vi "Init_Camera.vi"(4 "Binning IN":u32, 6 "Use Cursors IN":bool, 8 "Image Handle IN":u32=99 caption="Image Handle", 9 "ROI Parameters":T2={"X start"=1, "X end"=1340, "X Binning/Grouping"=1, "Y start"=1, "Y end"=400, "Y Binning/Grouping"=1}, 10 "integration time [s]":dbl=0.5, 11 "Parameters IN":T1={"camera parameters"={"Camera Handle"=16842752, "Xdim"=1340, "Ydim"=400}, "error"={"status"=FALSE, "code"=0, "source"=""}, "Plot height [pixel]"=0.0, "Plot width [pixel]"=0.0}) -> (0 "Image Handle OUT":u32 caption="Image Handle", 3 "Parameters OUT":T1={"camera parameters"={"Camera Handle"=16842752, "Xdim"=1340, "Ydim"=400}, "error"={"status"=FALSE, "code"=0, "source"=""}, "Plot height [pixel]"=0.0, "Plot width [pixel]"=0.0})   [LabVIEW 2013]
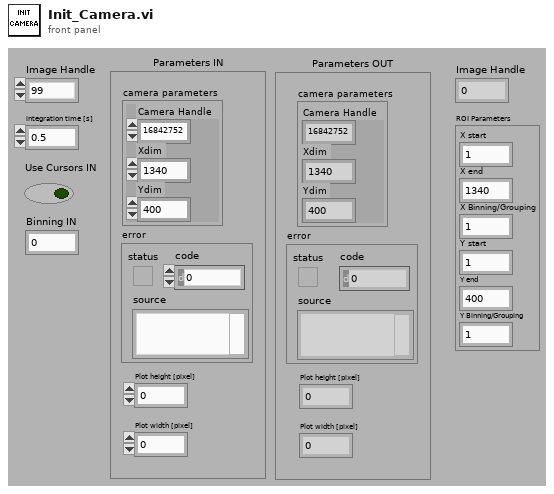
[diagram p1: front panel]
types:
  T1 = cluster{"camera parameters":cluster{"Camera Handle":u32, "Xdim":u32, "Ydim":u32}, "error":errorcluster, "Plot height [pixel]":dbl, "Plot width [pixel]":dbl}
  T2 = cluster{"X start":u32, "X end":u32, "X Binning/Grouping":u32, "Y start":u32, "Y end":u32, "Y Binning/Grouping":u32}
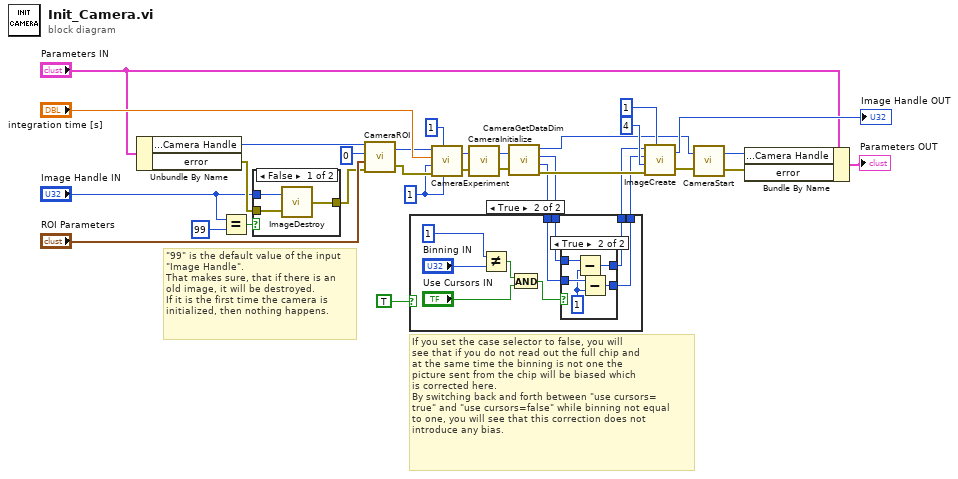
[diagram p0: block diagram]
diagram:
  w15 = 1
  # "If you set the case selector to false, you will\nsee that if you do not read out the full chip and\nat the same time the binning is not one the \npicture sent from the chip will be biased which\nis corrected here.\nBy switching back and forth between \"use cursors=\ntrue\" and \"use cursors=false\" while binning not equal\nto one, you will see that this correction does not\nintroduce any bias."
  # "\"99\" is the default value of the input\n\"Image Handle\".\nThat makes sure, that if there is an\nold image, it will be destroyed.\nIf it is the first time the camera is \ninitialized, then nothing happens."
  n1 = Unbundle By Name("Parameters IN") -> ("camera parameters.Camera Handle"=w31:u32, "error"=w9:errorcluster)
  n2 = Equal?(x="Image Handle IN", y=u32 99) -> (x = y?=w6:bool)
  n3 = case shown="False" w6 {
    tunnel: "Image Handle IN" -> [w35 _]
    tunnel: w9 -> [w34 w36]
    tunnel: [w33 w36] -> w10
    frame False {
      n4 = call <userlib>:"ImageDestroy.vi"("error in"=w34, "Data handle"=w35) -> ("error out"=w33:errorcluster)
    }
    frame True {
    }
  }
  n5 = call <userlib>:"CameraROI.vi"("error in"=w10, "ROI Params"="ROI Parameters", "ROI Index"=u32 0, "Camera Handle"=w31) -> ("error out"=w16:errorcluster, "Camera Handle"=w17:u32)
  n6 = call <userlib>:"CameraExperiment.vi"("Number of Accumulations"=w15, "Acquire / Focus Flag"=u32 1, "error in"=w16, "Number of Images"=w15, "Exposure (sec)"="integration time [s]", "Camera Handle"=w17) -> ("error out"=w20:errorcluster, "Camera Handle"=w21:u32)
  n7 = call <userlib>:"CameraInitialize.vi"("error in"=w20, "Camera Handle"=w21) -> ("error out"=w18:errorcluster, "Camera Handle"=w19:u32)
  n8 = call <userlib>:"CameraGetDataDim.vi"("Camera Handle"=w19, "error in"=w18) -> ("Camera Handle"=w12:u32, "Xdim"=w5:u32, "Ydim"=w4:u32, "error out"=w23:errorcluster)
  n9 = case shown="True" TRUE {
    tunnel: w5 -> [w38 w45]
    tunnel: w4 -> [w37 w44]
    tunnel: [w38 w43] -> w3
    tunnel: [w37 w42] -> w2
    frame False {
    }
    frame True {
      n10 = Not Equal?(x=u32 1, y="Binning IN") -> (x != y?=w41:bool)
      n11 = And(x=w41, y="Use Cursors IN") -> (x .and. y?=w40:bool)
      n12 = case shown="True" w40 {
        tunnel: w45 -> [w49 w51]
        tunnel: w44 -> [w48 w52]
        tunnel: [w49 w54] -> w43
        tunnel: [w48 w53] -> w42
        frame False {
        }
        frame True {
          w50 = u32 1 ("y")
          n13 = Subtract(x=w51, y=w50) -> (x-y=w54:u32)
          n14 = Subtract(x=w52, y=w50) -> (x-y=w53:u32)
        }
      }
    }
  }
  n15 = call <userlib>:"ImageCreate.vi"("X dimension"=w3, "Y dimension"=w2, "Data Type"=u32 4, "error in"=w23, "Number Of Frames"=u32 1) -> ("Image Handle"=→"Image Handle OUT":u32, "error out"=w13:errorcluster)
  n16 = call <userlib>:"CameraStart.vi"("error in"=w13, "Camera Handle"=w12) -> ("error out"=w27:errorcluster, "Camera Handle"=w26:u32)
  n17 = Bundle By Name(cluster="Parameters IN", "camera parameters.Camera Handle"=w26, "error"=w27) -> (→"Parameters OUT":T1)
